vi "ModifyGraph grid.vi"(8 "error in (no error)":errorcluster, 10 "Grid":T1, 11 "ITX Commands in":refnum<class "ITX Commands.lvclass">) -> (0 "error out":errorcluster, 3 "ITX Commands out":refnum<class "ITX Commands.lvclass">)   [LabVIEW 2016, in "ITX Commands.lvclass"]
uses:
  ITX Commands.lvclass
  typedefs/grid--enum.ctl
  ITX Commands.lvclass/ITX Commands.ctl
panel:
  out "resulting string":string
  # "g=0: Grid off. \ng=1: Grid on. \ng=2: Grid on major ticks only"
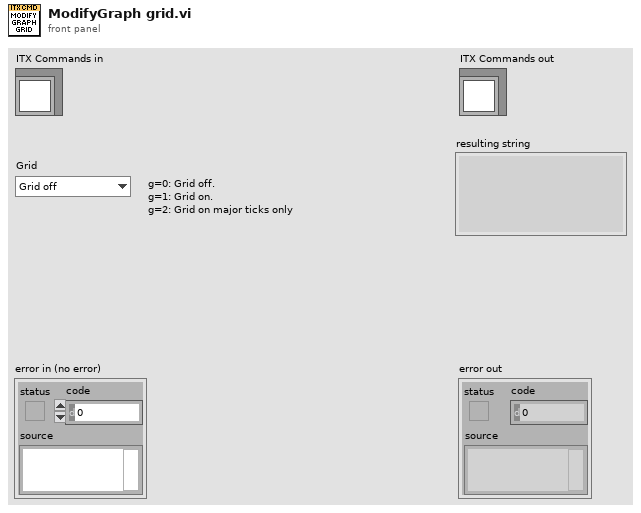
[diagram p1: front panel]
types:
  T1 = typedef "ITX Commands.lvclass/grid--enum.ctl" = enum16{"Grid off", "Grid on", "Grid on major ticks only"}
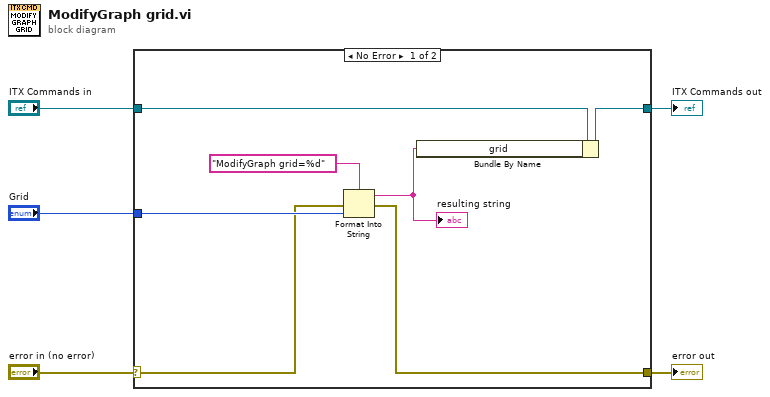
[diagram p0: block diagram]
diagram:
  n1 = case shown="No Error" "error in (no error)" {
    selector: "error in (no error)" -> [w7 w14]
    tunnel: [w6 w14] -> w4
    tunnel: [w8 w13] -> w2
    tunnel: "ITX Commands in" -> [w12 w13]
    tunnel: "Grid" -> [w9 _]
    frame No Error {
      n2 = Format Into String(format string="ModifyGraph grid=%d", error in=w7, w9) -> (resulting string=w10:string, error out=w6:errorcluster)  [unwired: 1 in]
      "resulting string" <- w10
      n3 = Bundle By Name(cluster=w12, "grid"=w10) -> (w8:refnum<class "ITX Commands.lvclass">)
    }
    frame Error {
    }
  }
  "error out" <- w4
  "ITX Commands out" <- w2
